vi "相机标定-汇川机械手.vi"() -> ()   [LabVIEW 2016]
uses:
  <vilib>/userdefined/High Color/IMAQdx.ctl
  CalibrateSteps.ctl
  <vilib>/vision/driver/IMAQdx.llb/IMAQdx Acquisition Mode.ctl
  <vilib>/vision/driver/IMAQdx.llb/IMAQdx Buffer Number Mode.ctl
  <vilib>/Utility/config.llb/Write Key (Boolean).vi
  <vilib>/vision/driver/NI_Vision_Acquisition_Software.lvlib
  <vilib>/Utility/config.llb/NI_LVConfig.lvlib
panel:
  in  "记录抓取位置":bool
  out "机械手抓取Y":dbl
  out "机械手抓取X":dbl
  out "连接成功":bool
  in  "重新连接":bool
  in  "X轴偏移量":dbl=10000.0
  in  "Y轴偏移量":dbl=10000.0
  in  "确定按钮":bool
  out "机械手坐标X":dbl
  out "机械手坐标Y":dbl
  out "像素坐标X":dbl
  out "像素坐标Y":dbl
  in  "强制退出":bool
  out "Image":T1(plugin-control)
  in  "CalibrationPath":path
  in  "SessionSelect":T2
  out "停止标志":bool
  # "影像显示"
  # "参数设置"
  # "结果显示"
  # "记录Mark位置"
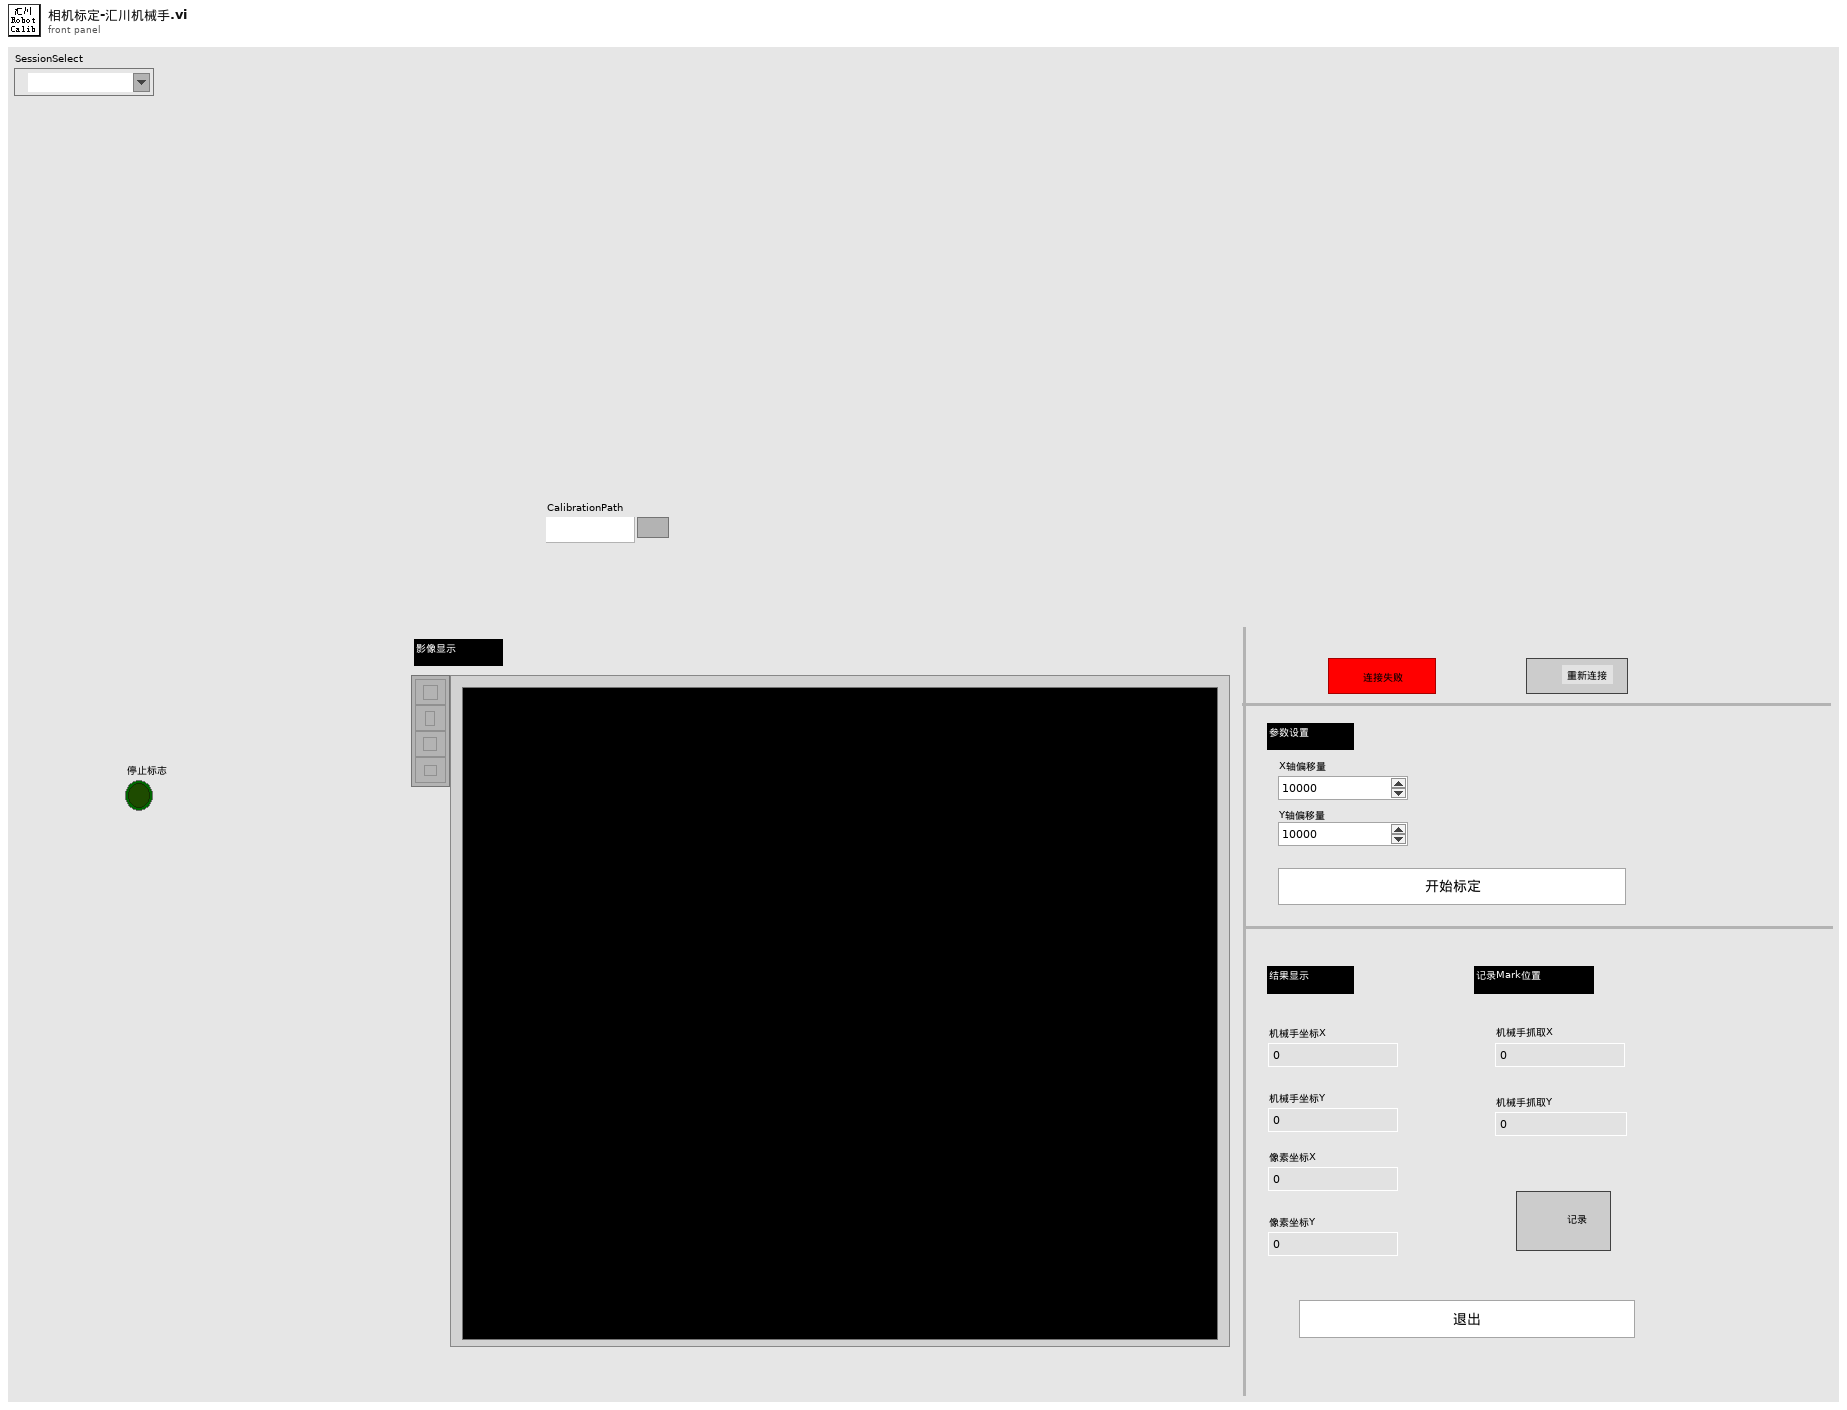
[diagram p1: front panel]
types:
  T1 = typedef "IMAQ Image.ctl" = refnum<image>
  T2 = typedef "IMAQdx.ctl" = refnum<k21>
  T3 = typedef "CalibrateSteps.ctl" = enum16{"初始化参数", "连接机械手", "连接相机", "机械手移动原位", "相机一次采集", "Y轴移动负偏移", "Y轴移动正偏移", "X轴移动正偏移", "X轴移动负偏移", "数据保存", "退出"}
  T4 = typedef "NI_LVConfig.lvlib/Config Data RefNum.ctl" = refnum<k1>
  T5 = enum16{"open", "replace", "create", "open or create", "replace or create", "replace or create with confirmation"}
  T6 = typedef "NI_Vision_Acquisition_Software.lvlib/IMAQdx Acquisition Mode.ctl" = enum32{"One Shot", "Continuous"}
  T7 = typedef "NI_Vision_Acquisition_Software.lvlib/IMAQdx Buffer Number Mode.ctl" = enum32{"Next", "Last", "Buffer Number", "Every", "Last New"}
  T8 = enum32{"Invalid", "Standard", "Closed", "Hidden", "Minimized", "Maximized"}
  T9 = cluster{"Center (Pixels)":cluster{"X":sgl, "Y":sgl}, "Radius (Pixels)":dbl, "Center (Real-World)":cluster{"X":sgl, "Y":sgl}, "Radius (Real-World)":dbl, "Roundness (Real-World)":dbl, "Average Strength":dbl, "Average SNR (dB)":dbl}
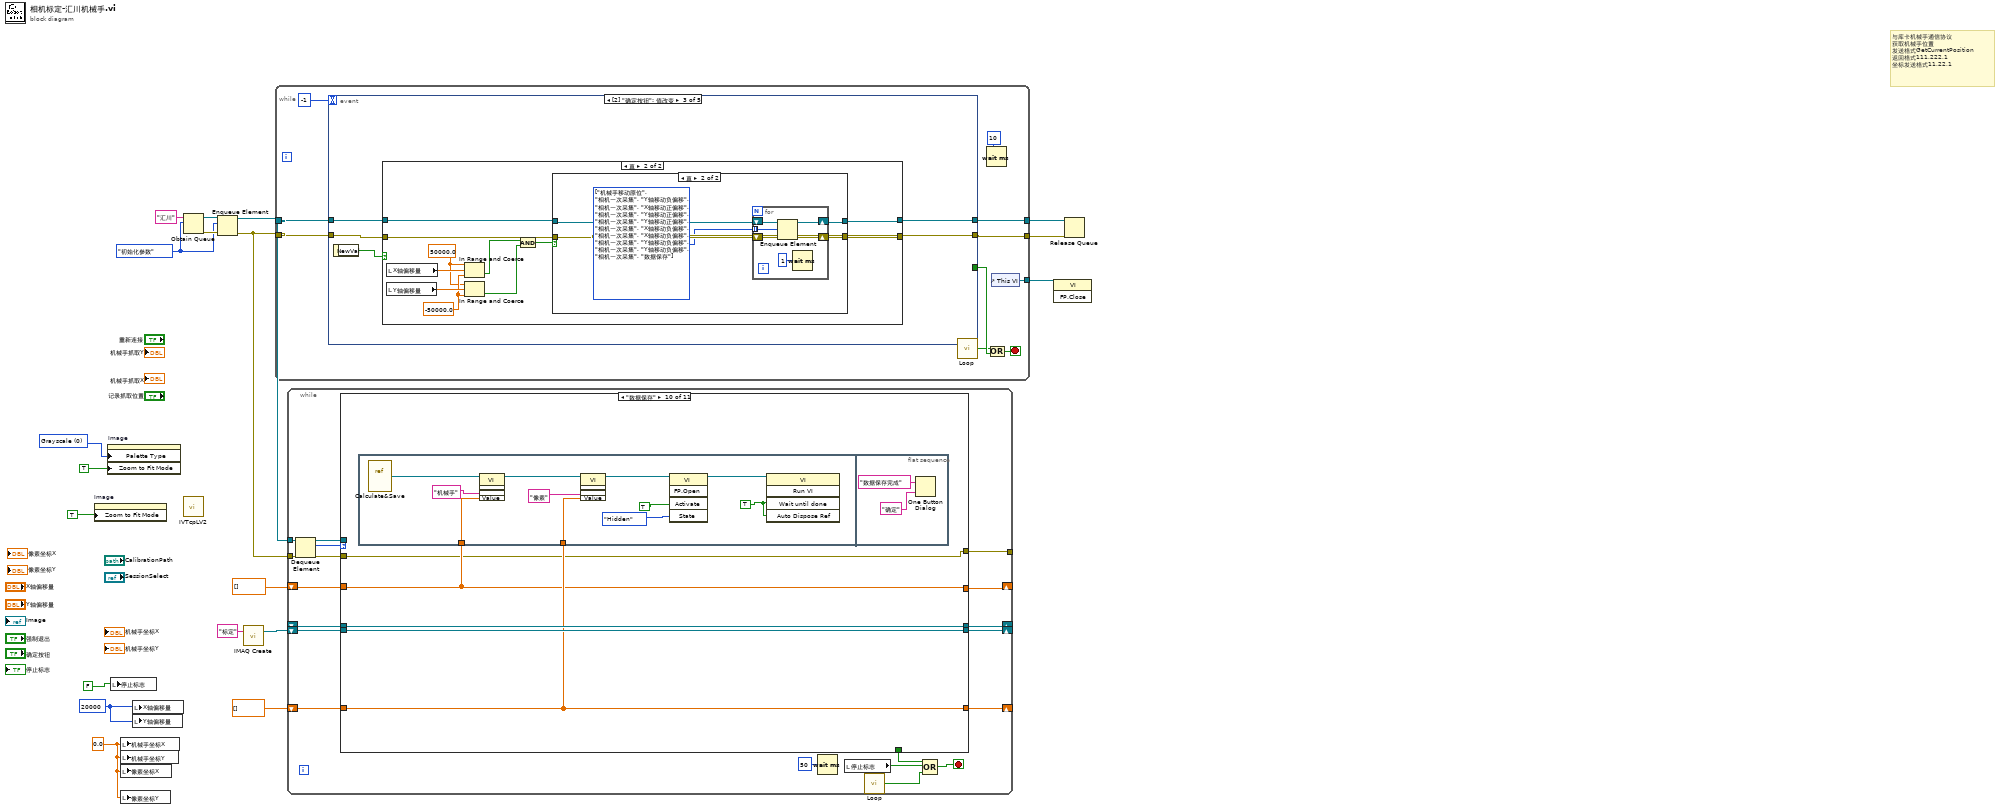
[diagram p0: block diagram]
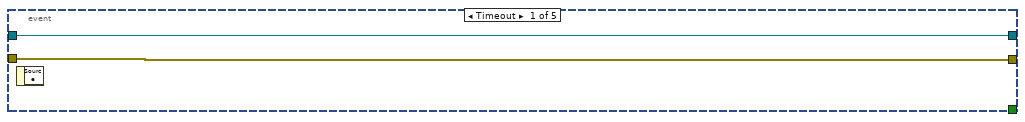
[diagram p2: hidden frame]
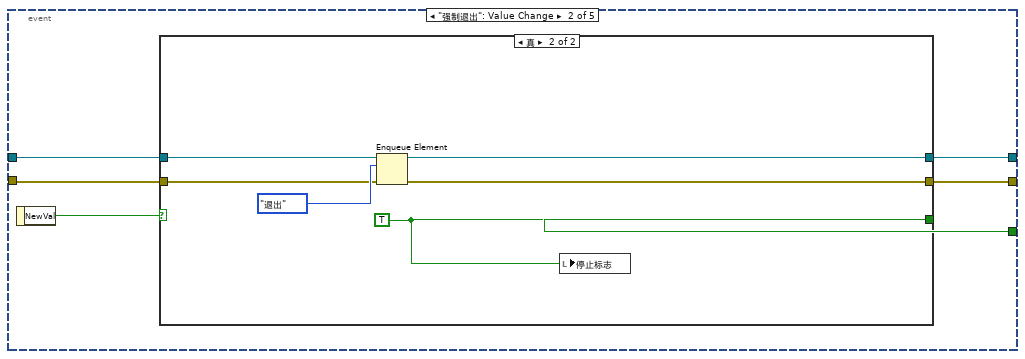
[diagram p3: hidden frame]
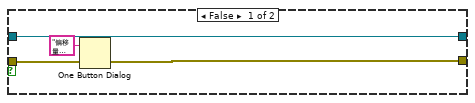
[diagram p6: hidden frame]
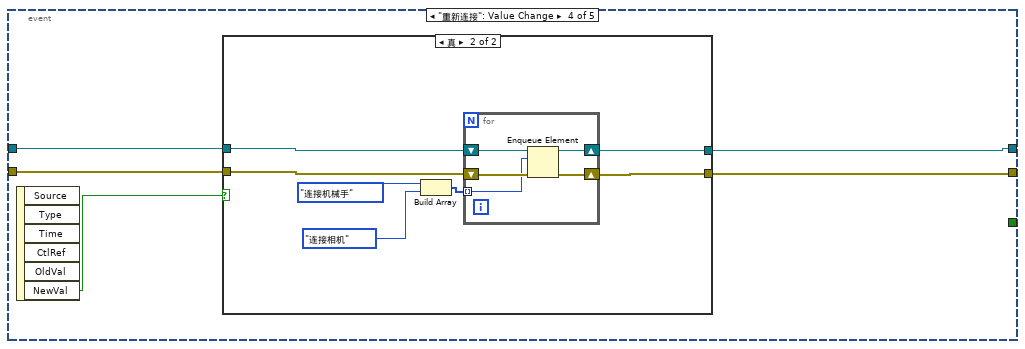
[diagram p7: hidden frame]
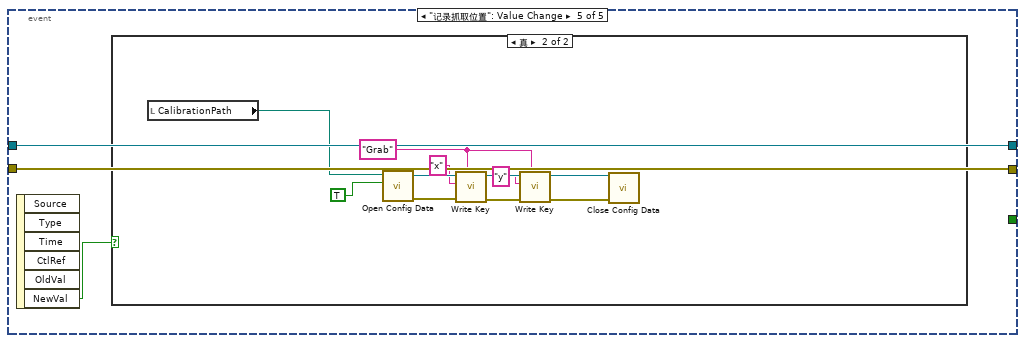
[diagram p9: hidden frame]
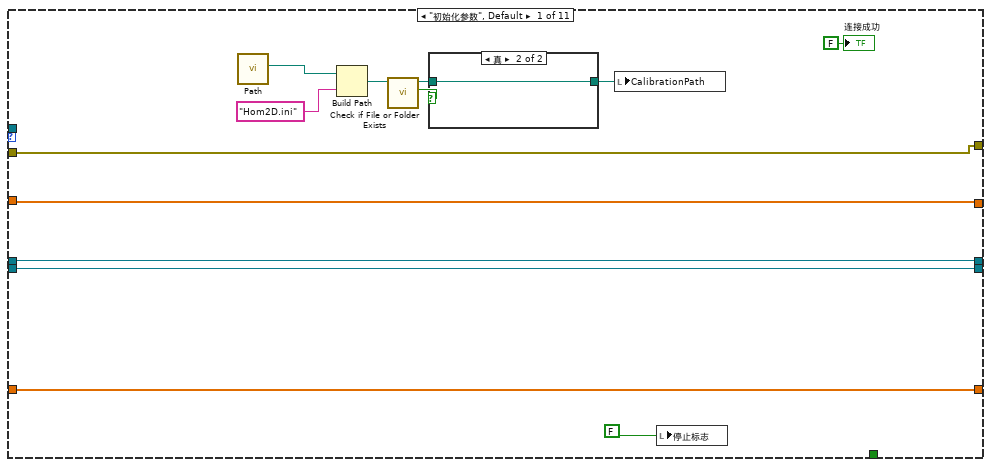
[diagram p11: hidden frame]
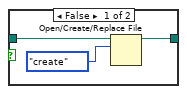
[diagram p12: hidden frame]
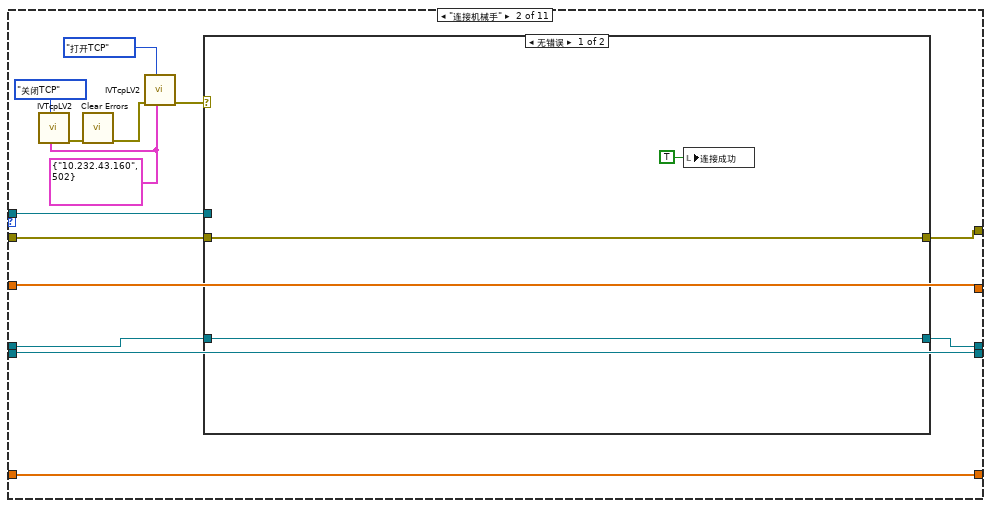
[diagram p13: hidden frame]
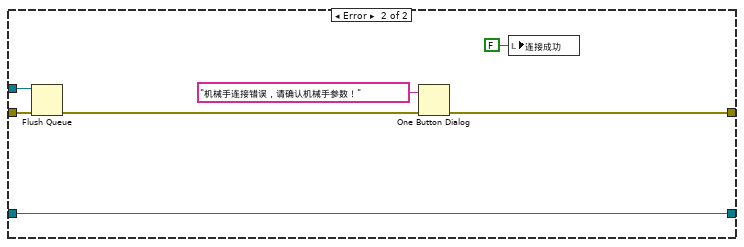
[diagram p14: hidden frame]
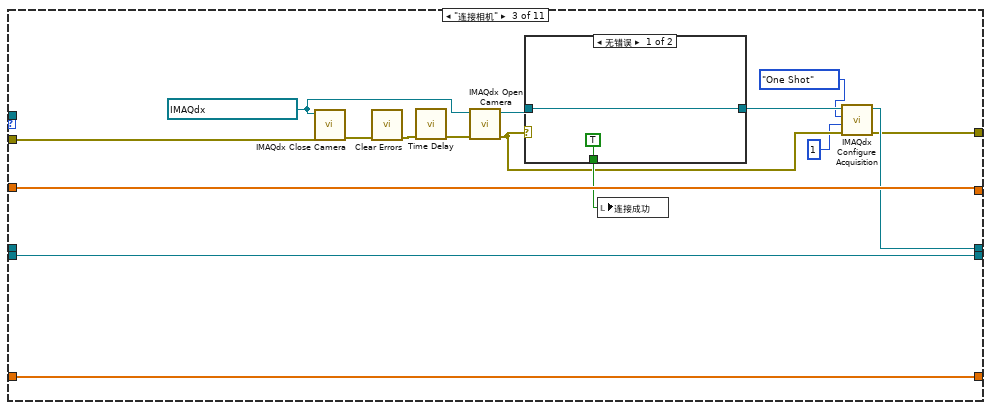
[diagram p15: hidden frame]
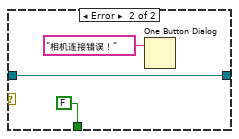
[diagram p16: hidden frame]
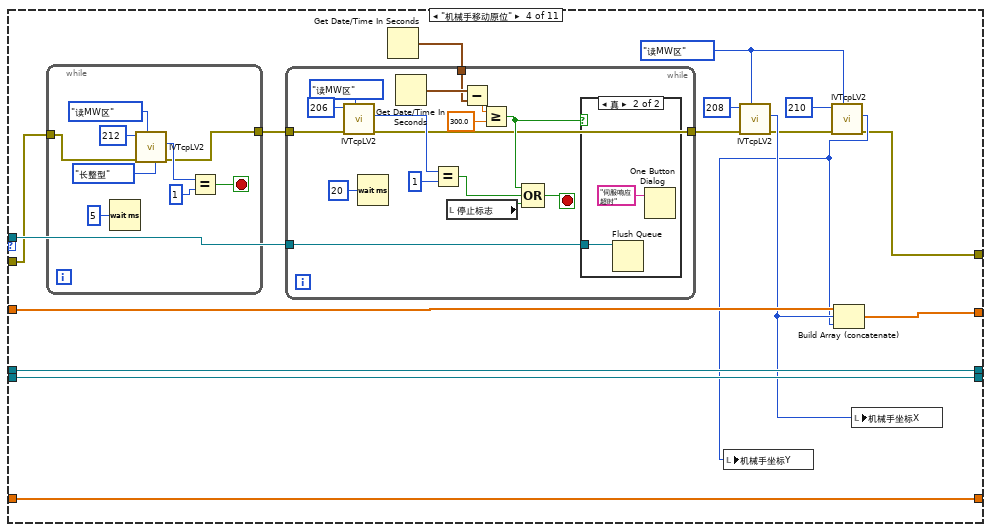
[diagram p17: hidden frame]
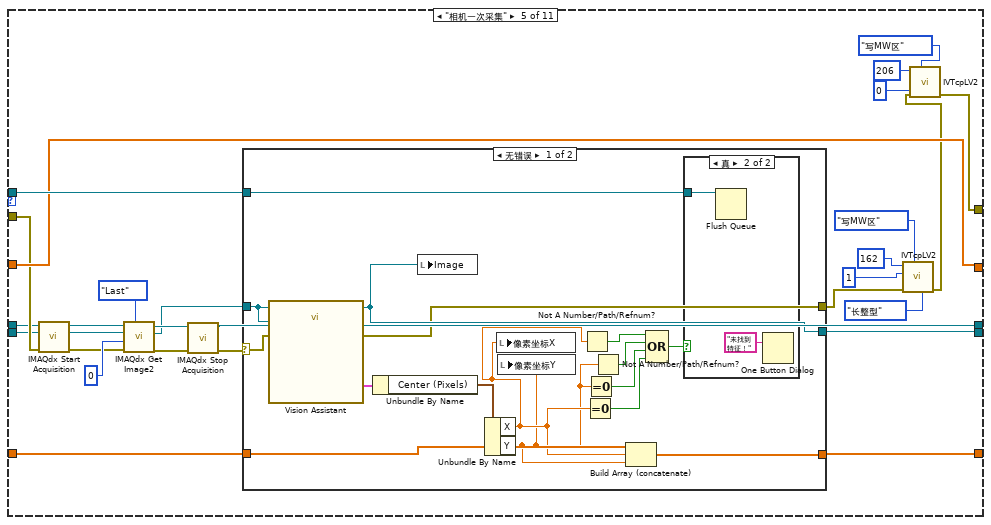
[diagram p19: hidden frame]
diagram:
  w3 = CalibrateSteps."初始化参数"
  w19 = 0.0 ("机械手当前X坐标")
  w16 = 20000
  w14 = u32 0 items=["Grayscale", "Binary", "Gradient", "Rainbow", "Temperature", "User Defined", "Binary 16 Bit", "Gradient 16 Bit", "Rainbow 16 Bit", "Temperature 16 Bit", "User Defined 16 Bit"] ("Palette:Palette Type")
  # "与库卡机械手通信协议\n获取机械手位置\n发送格式GetCurrentPosition\n返回格式111,222,1\n坐标发送格式11,22,1"
  n1 = property on="Image" class="ImageControl"("Zoom to Fit Mode"=TRUE) -> ()  [unwired: 2 in, 2 out]
  n2 = property on="Image" class="ImageControl"("Palette Type"=w14, "Zoom to Fit Mode"=TRUE) -> ()  [unwired: 2 in, 2 out]
  n3 = local write "停止标志"(FALSE ("停止标志")) -> ()
  n4 = local write "机械手坐标X"(w19) -> ()
  n5 = local write "机械手坐标Y"(w19) -> ()
  n6 = local write "像素坐标X"(w19) -> ()
  n7 = local write "像素坐标Y"(w19) -> ()
  n8 = local write "X轴偏移量"(w16) -> ()
  n9 = local write "Y轴偏移量"(w16) -> ()
  n10 = Obtain Queue(name (unnamed)="汇川", element data type=w3) -> (queue out=w6:refnum<queue>, error out=w5:errorcluster)  [unwired: 3 in, 1 out]
  n11 = call "IVTcpLV2.vi"() -> ()  [unwired: 8 in, 4 out]
  n12 = Enqueue Element(queue=w6, element=w3, error in (no error)=w5) -> (queue out=w4:refnum<queue>, error out=w2:errorcluster)  [unwired: 1 in, 1 out]
  n13 = call "IMAQ Create"("Image Name"="标定") -> ("New Image"=w8:T1)  [unwired: 4 in, 1 out]
  n14 = while {
    tunnel: w4 -> [w29]
    tunnel: w2 -> [w28]
    tunnel: [w27] -> w11
    tunnel: [w26] -> w12
    tunnel: [w24] -> w13
    stop <- w23 stop-if-true
    n15 = event shown="[2] \"确定按钮\": 值改变" {
      selector: _ -> [_ _ _ _ _]
      dyn-events: _ -> [_ _ _ _ _]
      timeout: -1 -> [_ _ _ _ _]
      tunnel: w29 -> [w31 w36 w49 w79 w98]
      tunnel: w28 -> [w30 w33 w48 w78 w97]
      tunnel: [w31 w35 w47 w81 w98] -> w27
      tunnel: [w30 w32 w46 w80 w97] -> w26
      tunnel: [_ w34 _ _ _] -> w22
      event Timeout {
        n16 = event-data() -> ()  [unwired: 1 in, 1 out]
      }
      event "强制退出": Value Change {
        n17 = event-data() -> ("NewVal"=w37:bool)  [unwired: 1 in]
        n18 = case shown="真" w37 {
          tunnel: [_ w43] -> w34
          tunnel: w36 -> [w39 w45]
          tunnel: [w39 w44] -> w35
          tunnel: w33 -> [w38 w41]
          tunnel: [w38 w40] -> w32
          frame False {
          }
          frame True {
            w43 = TRUE
            n19 = Enqueue Element(queue=w45, element=CalibrateSteps."退出", error in (no error)=w41) -> (queue out=w44:refnum<queue>, error out=w40:errorcluster)  [unwired: 1 in, 1 out]
            n20 = local write "停止标志"(w43) -> ()
          }
        }
      }
      event "确定按钮": Value Change {
        n21 = event-data() -> ("NewVal"=w50:bool)  [unwired: 1 in]
        n22 = case shown="真" w50 {
          tunnel: w49 -> [w52 w54]
          tunnel: w48 -> [w51 w53]
          tunnel: [w52 w56] -> w47
          tunnel: [w51 w55] -> w46
          frame False {
          }
          frame True {
            w58 = -50000.0 ("下限")
            w57 = 50000.0 ("上限")
            n23 = local read "Y轴偏移量"() -> (w60:dbl)
            n24 = local read "X轴偏移量"() -> (w59:dbl)
            n25 = In Range and Coerce(upper limit=w57, x=w60, lower limit=w58) -> (In Range?=w62:bool)  [unwired: 1 out]
            n26 = In Range and Coerce(upper limit=w57, x=w59, lower limit=w58) -> (In Range?=w61:bool)  [unwired: 1 out]
            n27 = And(x=w61, y=w62) -> (x .and. y?=w63:bool)
            n28 = case shown="真" w63 {
              tunnel: [w65 w71] -> w56
              tunnel: [w64 w70] -> w55
              tunnel: w54 -> [w65 w69]
              tunnel: w53 -> [w64 w68]
              frame False {
                n29 = One Button Dialog(message="偏移量设置太大请重新设置！" ("消息")) -> ()  [unwired: 1 in, 1 out]
              }
              frame True {
                w67 = T3[] [enum."机械手移动原位", enum."相机一次采集", enum."Y轴移动负偏移", enum."相机一次采集", enum."X轴移动正偏移", enum."相机一次采集", enum."Y轴移动正偏移", enum."相机一次采集", enum."Y轴移动正偏移", enum."相机一次采集", enum."X轴移动负偏移", enum."相机一次采集", enum."X轴移动负偏移", enum."相机一次采集", enum."Y轴移动负偏移", enum."相机一次采集", enum."Y轴移动负偏移", enum."相机一次采集", enum."数据保存"] items=["初始化参数", "连接机械手", "连接相机", "机械手移动原位", "相机一次采集", "Y轴移动负偏移", "Y轴移动正偏移", "X轴移动正偏移", "X轴移动负偏移", "数据保存", "退出"] ("Array")
                n30 = for {
                  shift-right: [w75] -> w71
                  shift-left: w69 -> [w77]
                  shift-right: [w74] -> w70
                  shift-left: w68 -> [w76]
                  tunnel: w67 -> [w73] mode=indexing
                  n31 = Enqueue Element(queue=w77, element=w73, error in (no error)=w76) -> (queue out=w75:refnum<queue>, error out=w74:errorcluster)  [unwired: 1 in, 1 out]
                  n32 = Wait (ms)(milliseconds to wait=u32 1 ("等待时间（毫秒）")) -> ()  [unwired: 1 out]
                }
              }
            }
          }
        }
      }
      event "重新连接": Value Change {
        n33 = event-data() -> ("NewVal"=w82:bool)  [unwired: 1 in, 5 out]
        n34 = case shown="真" w82 {
          tunnel: [w84 w91] -> w81
          tunnel: [w83 w90] -> w80
          tunnel: w79 -> [w84 w89]
          tunnel: w78 -> [w83 w88]
          frame False {
          }
          frame True {
            n35 = Build Array(CalibrateSteps."连接机械手", CalibrateSteps."连接相机") -> (w87:T3[])
            n36 = for {
              shift-right: [w94] -> w91
              shift-left: w89 -> [w96]
              shift-right: [w93] -> w90
              shift-left: w88 -> [w95]
              tunnel: w87 -> [w92] mode=indexing
              n37 = Enqueue Element(queue=w96, element=w92, error in (no error)=w95) -> (queue out=w94:refnum<queue>, error out=w93:errorcluster)  [unwired: 1 in, 1 out]
            }
          }
        }
      }
      event "记录抓取位置": Value Change {
        n38 = event-data() -> ("NewVal"=w99:bool)  [unwired: 1 in, 5 out]
        n39 = case shown="真" w99 {
          frame False {
          }
          frame True {
            w105 = "Grab" ("key")
            n40 = local read "CalibrationPath"() -> (w102:path)
            n41 = call <vilib>:"Open Config Data.vi"("create file if necessary (T)"=TRUE, "configuration file path"=w102) -> ("error out"=w108:errorcluster, "refnum"=w110:T4)  [unwired: 7 in, 1 out]
            n42 = call-poly <vilib>:"Write Key.vi"("section"=w105, "error in (no error)"=w108, "key"="x", "refnum"=w110) -> ("error out"=w107:errorcluster, "refnum out"=w106:T4)  [unwired: 5 in, 1 out]
            n43 = call-poly <vilib>:"Write Key.vi"("section"=w105, "error in (no error)"=w107, "key"="y", "refnum"=w106) -> ("error out"=w100:errorcluster, "refnum out"=w101:T4)  [unwired: 5 in, 1 out]
            n44 = call <vilib>:"Close Config Data.vi"("error in (no error)"=w100, "refnum"=w101) -> ()  [unwired: 8 in, 2 out]
          }
        }
      }
    }
    n45 = call "Loop.vi"() -> ("Loop Out"=w21:bool)  [unwired: 5 in]
    n46 = Wait (ms)(milliseconds to wait=u32 10 ("等待时间（毫秒）")) -> ()  [unwired: 1 out]
    n47 = Compound Arithmetic op=OR ("复合运算")(w21, w22) -> (w23:bool)
    n48 = control-ref of="This VI"() -> (w24:refnum<vi>)
  }
  n49 = while {
    shift-right: [w126] -> _
    shift-left: dbl[] [] -> [w125]
    shift-right: [w116] -> _
    shift-left: dbl[] [] -> [w112]
    shift-right: [w123] -> _
    shift-left: _ -> [w122]
    shift-right: [w120] -> _
    shift-left: w8 -> [w121]
    tunnel: w4 -> [w119]
    tunnel: w2 -> [w115]
    tunnel: [w113] -> _
    stop <- w127 stop-if-true
    n50 = Dequeue Element(queue=w119, error in (no error)=w115) -> (queue out=w117:refnum<queue>, element=w118:T3, error out=w114:errorcluster)  [unwired: 1 in, 1 out]
    n51 = case shown="\"数据保存\"" w118 {
      tunnel: w112 -> [w139 w155 w184 w206 w256 w309 w346 w390 w432 w455 w472]
      tunnel: [w139 w155 w184 w204 w256 w306 w345 w389 w431 w455 w472] -> w116
      tunnel: [w142 w159 w169 w205 w260 w310 w344 w385 w427 w456 w477] -> w126
      tunnel: w125 -> [w142 w159 w169 w205 w259 w310 w344 w385 w427 w456 w477]
      tunnel: [_ _ _ _ _ _ _ _ _ _ TRUE] -> w124
      tunnel: [w141 w158 w173 w203 w249 w308 w352 w394 w436 w458 w476] -> w123
      tunnel: w122 -> [w141 w157 _ w203 w246 w308 w352 w394 w436 w458 w476]
      tunnel: [w140 w156 w183 w202 w258 w307 w351 w393 w435 w457 w475] -> w120
      tunnel: w121 -> [w140 w156 w183 w202 w251 w307 w351 w393 w435 w457 w475]
      tunnel: w117 -> [_ w154 _ w200 w257 w303 w348 w388 w430 _ _]
      tunnel: w114 -> [w131 w153 w175 w199 w253 w295 w347 w378 w420 w454 w473]
      tunnel: [w131 w152 w172 w190 w235 w293 w347 w377 w420 w454 w473] -> w113
      frame "初始化参数", Default {
        n52 = call "Path.vi"() -> ("Total"=w130:path)  [unwired: 11 in]
        n53 = Build Path(base path=w130, name or relative path="Hom2D.ini") -> (appended path=w136:path)
        n54 = call <vilib>:"Check if File or Folder Exists.vi"("path"=w136) -> ("file or folder exists?"=w138:bool, "dup path"=w137:path)  [unwired: 8 in, 1 out]
        n55 = case shown="真" w138 {
          tunnel: w137 -> [w144 w145]
          tunnel: [w144 w145] -> w135
          frame False {
            n56 = Open/Create/Replace File(file path (use dialog)=w144, operation (0:open)=T5."create") -> ()  [unwired: 4 in, 3 out]
          }
          frame True {
          }
        }
        n57 = local write "CalibrationPath"(w135) -> ()
        n58 = local write "停止标志"(FALSE ("停止标志")) -> ()
        "连接成功" <- FALSE ("连接成功")
      }
      frame "连接机械手" {
        w146 = cluster{"IP地址":string, "端口":u16} {"IP地址"="10.232.43.160", "端口"=502} ("TCP连接参数")
        n59 = call "IVTcpLV2.vi"("TCP连接参数"=w146, "TCP操作模式"=enum16{"打开TCP", "读MW区", "写MW区", "关闭TCP"}."关闭TCP") -> ("错误输出"=w147:errorcluster)  [unwired: 6 in, 3 out]
        n60 = call <vilib>:"Clear Errors.vi"("error in (no error)"=w147) -> ("error out"=w151:errorcluster)  [unwired: 5 in, 1 out]
        n61 = call "IVTcpLV2.vi"("TCP连接参数"=w146, "TCP操作模式"=enum16{"打开TCP", "读MW区", "写MW区", "关闭TCP"}."打开TCP", "错误输入"=w151) -> ("错误输出"=w150:errorcluster)  [unwired: 5 in, 3 out]
        n62 = case shown="无错误" w150 {
          tunnel: [w162 w168] -> w158
          tunnel: w157 -> [w162 w168]
          tunnel: w154 -> [_ w166]
          tunnel: w153 -> [w160 w164]
          tunnel: [w160 w163] -> w152
          frame No Error {
            n63 = local write "连接成功"(TRUE ("连接成功")) -> ()
          }
          frame Error {
            n64 = Flush Queue(queue=w166, error in (no error)=w164) -> (error out=w163:errorcluster)  [unwired: 2 out]
            n65 = One Button Dialog(message="机械手连接错误，请确认机械手参数！") -> ()  [unwired: 1 in, 1 out]
            n66 = local write "连接成功"(FALSE ("连接成功")) -> ()
          }
        }
      }
      frame "连接相机" {
        w177 = T2 "MV-CA060-11GM" ("Session In")
        n67 = call <vilib>:"IMAQdx Close Camera.vi"("error in"=w175, "Session In"=w177) -> ("error out"=w182:errorcluster)  [unwired: 9 in]
        n68 = call <vilib>:"Clear Errors.vi"("error in (no error)"=w182) -> ("error out"=w181:errorcluster)  [unwired: 5 in, 1 out]
        n69 = call "Time Delay"("error in (no error)"=w181) -> ("error out"=w180:errorcluster)  [unwired: 10 in]
        n70 = call <vilib>:"IMAQdx Open Camera.vi"("error in"=w180, "Session In"=w177) -> ("error out"=w174:errorcluster, "Session Out"=w179:T2)  [unwired: 8 in]
        n71 = case shown="无错误" w174 {
          tunnel: w179 -> [w186 w189]
          tunnel: [w186 w189] -> w176
          tunnel: [TRUE ("连接成功") FALSE ("连接成功")] -> w178
          frame No Error {
          }
          frame Error {
            n72 = One Button Dialog(message="相机连接错误！") -> ()  [unwired: 1 in, 1 out]
          }
        }
        n73 = local write "连接成功"(w178) -> ()
        n74 = call <vilib>:"IMAQdx Configure Acquisition.vi"("error in"=w174, "Number of Buffers"=u32 1, "Continuous?"=IMAQdx_Acquisition_Mode."One Shot", "Session In"=w176) -> ("error out"=w172:errorcluster, "Session Out"=w173:T2)  [unwired: 6 in]
      }
      frame "机械手移动原位" {
        w193 = enum16{"打开TCP", "读MW区", "写MW区", "关闭TCP"}."读MW区" ("TCP操作模式")
        n75 = while {
          tunnel: w199 -> [w212]
          tunnel: [w207] -> w198
          stop <- w210 stop-if-true
          n76 = Wait (ms)(milliseconds to wait=u32 5 ("等待时间（毫秒）")) -> ()  [unwired: 1 out]
          n77 = call "IVTcpLV2.vi"("数值类型"=enum16{"长整型", "双精度"}."长整型", "TCP操作模式"=enum16{"打开TCP", "读MW区", "写MW区", "关闭TCP"}."读MW区", "错误输入"=w212, "寄存器MD地址"=212) -> ("错误输出"=w207:errorcluster, "数值"=w211:u32)  [unwired: 4 in, 2 out]
          n78 = Equal?(x=w211, y=1) -> (x = y?=w210:bool)
        }
        n79 = Get Date/Time In Seconds() -> (seconds since 1Jan1904=w201:timestamp)
        n80 = while {
          tunnel: w198 -> [w223]
          tunnel: w201 -> [w226]
          tunnel: w200 -> [w224]
          tunnel: [w216] -> w197
          stop <- w231 stop-if-true
          n81 = call "IVTcpLV2.vi"("TCP操作模式"=enum16{"打开TCP", "读MW区", "写MW区", "关闭TCP"}."读MW区", "错误输入"=w223, "寄存器MD地址"=206) -> ("错误输出"=w216:errorcluster, "数值"=w219:u32)  [unwired: 5 in, 2 out]
          n82 = Wait (ms)(milliseconds to wait=u32 20 ("等待时间（毫秒）")) -> ()  [unwired: 1 out]
          n83 = Get Date/Time In Seconds() -> (seconds since 1Jan1904=w228:timestamp)
          n84 = Equal?(x=w219, y=u32 1) -> (x = y?=w217:bool)
          n85 = local read "停止标志"() -> (w230:bool)
          n86 = Subtract(x=w228, y=w226) -> (x-y=w229:dbl)
          n87 = Greater Or Equal?(x=w229, y=300.0) -> (x >= y?=w225:bool)
          n88 = Compound Arithmetic op=OR(w225, w217, w230) -> (w231:bool)
          n89 = case shown="真" w225 {
            tunnel: w224 -> [_ w232]
            frame False {
            }
            frame True {
              n90 = Flush Queue(queue=w232) -> ()  [unwired: 1 in, 3 out]
              n91 = One Button Dialog(message="伺服响应超时") -> ()  [unwired: 1 in, 1 out]
            }
          }
        }
        n92 = call "IVTcpLV2.vi"("TCP操作模式"=w193, "错误输入"=w197, "寄存器MD地址"=208) -> ("错误输出"=w194:errorcluster, "数值"=w195:u32)  [unwired: 5 in, 2 out]
        n93 = call "IVTcpLV2.vi"("TCP操作模式"=w193, "错误输入"=w194, "寄存器MD地址"=210) -> ("错误输出"=w190:errorcluster, "数值"=w191:u32)  [unwired: 5 in, 2 out]
        n94 = local write "机械手坐标Y"(w191) -> ()
        n95 = Build Array (concatenate)(w206, w195, w191) -> (w204:dbl[])
        n96 = local write "机械手坐标X"(w195) -> ()
      }
      frame "相机一次采集" {
        n97 = call <vilib>:"IMAQdx Start Acquisition.vi"("error in"=w253, "Session In"=w246) -> ("error out"=w247:errorcluster, "Session Out"=w252:T2)  [unwired: 8 in]
        n98 = call <vilib>:"IMAQdx Get Image2.vi"("Buffer Number Mode (Next)"=IMAQdx_Buffer_Number_Mode."Last", "error in"=w247, "Buffer Number In"=u32 0, "Image In"=w251, "Session In"=w252) -> ("error out"=w248:errorcluster, "Image Out"=w244:T1, "Session Out"=w250:T2)  [unwired: 3 in, 1 out]
        n99 = call <vilib>:"IMAQdx Stop Acquisition.vi"("error in"=w248, "Session In"=w250) -> ("error out"=w245:errorcluster, "Session Out"=w249:T2)  [unwired: 8 in]
        n100 = case shown="无错误" w245 {
          selector: w245 -> [w262 w279]
          tunnel: [w276 w285] -> w260
          tunnel: w259 -> [w275 w285]
          tunnel: [w263 w281] -> w258
          tunnel: w257 -> [w271 w282]
          tunnel: w244 -> [w268 w281]
          tunnel: [w261 w280] -> w243
          frame No Error {
            n101 = call "Vision Assistant"("Image In"=w268, "Image Dst"=w268, "error in"=w262) -> ("Image Out"=w263:T1, "Fitted Circle (Find Circular Edge 1)"=w267:T9, "error out"=w261:errorcluster)  [unwired: 22 in]
            n102 = Unbundle By Name(w267) -> ("Center (Pixels)"=w266:cluster{"X":sgl, "Y":sgl})
            n103 = local write "Image"(w263) -> ()
            n104 = Unbundle By Name(w266) -> ("X"=w265:sgl, "Y"=w264:sgl)
            n105 = local write "像素坐标X"(w265) -> ()
            n106 = local write "像素坐标Y"(w264) -> ()
            n107 = Not A Number/Path/Refnum?(number/path/refnum=w265) -> (NaN/Path/Refnum?=w273:bool)
            n108 = Equal To 0?(x=w265) -> (x = 0?=w269:bool)
            n109 = Equal To 0?(x=w264) -> (x = 0?=w270:bool)
            n110 = Not A Number/Path/Refnum?(number/path/refnum=w264) -> (NaN/Path/Refnum?=w272:bool)
            n111 = Build Array (concatenate)(w275, w265, w264) -> (w276:dbl[])
            n112 = Compound Arithmetic op=OR(w273, w272, w270, w269) -> (w274:bool)
            n113 = case shown="真" w274 {
              tunnel: w271 -> [_ w277]
              frame False {
              }
              frame True {
                n114 = Flush Queue(queue=w277) -> ()  [unwired: 1 in, 3 out]
                n115 = One Button Dialog(message="未找到特征！") -> ()  [unwired: 1 in, 1 out]
              }
            }
          }
          frame Error {
            n116 = Flush Queue(queue=w282) -> ()  [unwired: 1 in, 3 out]
            n117 = One Button Dialog(message="相机出错，检查相机连接！" ("消息"), button name ("OK")="确定" ("按钮名称（“确定”）")) -> ()  [unwired: 1 out]
            n118 = call <vilib>:"Clear Errors.vi"("error in (no error)"=w279) -> ("error out"=w280:errorcluster)  [unwired: 5 in, 1 out]
          }
        }
        n119 = call "IVTcpLV2.vi"("数值类型"=enum16{"长整型", "双精度"}."长整型", "TCP操作模式"=enum16{"打开TCP", "读MW区", "写MW区", "关闭TCP"}."写MW区", "错误输入"=w243, "值"=1, "寄存器MD地址"=162) -> ("错误输出"=w236:errorcluster)  [unwired: 3 in, 3 out]
        n120 = call "IVTcpLV2.vi"("TCP操作模式"=enum16{"打开TCP", "读MW区", "写MW区", "关闭TCP"}."写MW区", "错误输入"=w236, "值"=0, "寄存器MD地址"=206) -> ("错误输出"=w235:errorcluster)  [unwired: 4 in, 3 out]
      }
      frame "Y轴移动负偏移" {
        w291 = enum16{"打开TCP", "读MW区", "写MW区", "关闭TCP"}."写MW区" ("TCP操作模式")
        n121 = local read "机械手坐标X"() -> (w300:dbl)
        n122 = local read "机械手坐标Y"() -> (w302:dbl)
        n123 = local read "Y轴偏移量"() -> (w301:dbl)
        n124 = Subtract(x=w302, y=w301) -> (x-y=w299:dbl)
        n125 = Multiply(x=w301, y=-1.0) -> (x*y=w297:dbl)
        n126 = call "IVTcpLV2.vi"("TCP操作模式"=w291, "错误输入"=w295, "值"=w297, "寄存器MD地址"=138) -> ("错误输出"=w292:errorcluster)  [unwired: 4 in, 3 out]
        n127 = call "IVTcpLV2.vi"("TCP操作模式"=w291, "错误输入"=w292, "值"=0, "寄存器MD地址"=136) -> ("错误输出"=w288:errorcluster)  [unwired: 4 in, 3 out]
        n128 = local write "机械手坐标X"(w300) -> ()
        n129 = local write "机械手坐标Y"(w299) -> ()
        n130 = call "Time Delay3"("error in (no error)"=w288) -> ("error out"=w286:errorcluster)  [unwired: 10 in]
        n131 = call "IVTcpLV2.vi"("TCP操作模式"=w291, "错误输入"=w286, "值"=1, "寄存器MD地址"=160) -> ("错误输出"=w287:errorcluster)  [unwired: 4 in, 3 out]
        n132 = Get Date/Time In Seconds() -> (seconds since 1Jan1904=w304:timestamp)
        n133 = while {
          tunnel: w287 -> [w317]
          tunnel: w304 -> [w320]
          tunnel: w303 -> [w318]
          tunnel: [w311] -> w293
          stop <- w326 stop-if-true
          n134 = call "IVTcpLV2.vi"("TCP操作模式"=enum16{"打开TCP", "读MW区", "写MW区", "关闭TCP"}."读MW区", "错误输入"=w317, "寄存器MD地址"=206) -> ("错误输出"=w311:errorcluster, "数值"=w314:u32)  [unwired: 5 in, 2 out]
          n135 = Equal?(x=w314, y=u32 1) -> (x = y?=w312:bool)
          n136 = local read "停止标志"() -> (w324:bool)
          n137 = Wait (ms)(milliseconds to wait=u32 20 ("等待时间（毫秒）")) -> ()  [unwired: 1 out]
          n138 = Get Date/Time In Seconds() -> (seconds since 1Jan1904=w322:timestamp)
          n139 = Subtract(x=w322, y=w320) -> (x-y=w323:dbl)
          n140 = Greater Or Equal?(x=w323, y=300.0) -> (x >= y?=w319:bool)
          n141 = Compound Arithmetic op=OR(w319, w312, w324) -> (w326:bool)
          n142 = case shown="假" w319 {
            tunnel: w318 -> [_ w327]
            frame False {
            }
            frame True {
              n143 = Flush Queue(queue=w327) -> ()  [unwired: 1 in, 3 out]
              n144 = One Button Dialog(message="机械手响应超时") -> ()  [unwired: 1 in, 1 out]
            }
          }
        }
        n145 = Build Array (concatenate)(w309, w300, w299) -> (w306:dbl[])
      }
      frame "Y轴移动正偏移" {
        w334 = enum16{"打开TCP", "读MW区", "写MW区", "关闭TCP"}."写MW区" ("TCP操作模式")
        n146 = local read "机械手坐标Y"() -> (w343:dbl)
        n147 = local read "机械手坐标X"() -> (w341:dbl)
        n148 = local read "Y轴偏移量"() -> (w342:dbl)
        n149 = Add(x=w343, y=w342) -> (x+y=w340:dbl)
        n150 = Multiply(x=w342, y=1.0) -> (x*y=w336:dbl)
        n151 = call "IVTcpLV2.vi"("TCP操作模式"=w334, "值"=w336, "寄存器MD地址"=138) -> ("错误输出"=w335:errorcluster)  [unwired: 5 in, 3 out]
        n152 = local write "机械手坐标X"(w341) -> ()
        n153 = local write "机械手坐标Y"(w340) -> ()
        n154 = call "IVTcpLV2.vi"("TCP操作模式"=w334, "错误输入"=w335, "值"=0, "寄存器MD地址"=136) -> ("错误输出"=w330:errorcluster)  [unwired: 4 in, 3 out]
        n155 = call "Time Delay4"("error in (no error)"=w330) -> ("error out"=w329:errorcluster)  [unwired: 10 in]
        n156 = call "IVTcpLV2.vi"("TCP操作模式"=w334, "错误输入"=w329, "值"=1, "寄存器MD地址"=160) -> ("错误输出"=w331:errorcluster)  [unwired: 4 in, 3 out]
        n157 = Get Date/Time In Seconds() -> (seconds since 1Jan1904=w349:timestamp)
        n158 = while {
          tunnel: w331 -> [w356]
          tunnel: w349 -> [w361]
          tunnel: w348 -> [w359]
          stop <- w367 stop-if-true
          n159 = call "IVTcpLV2.vi"("TCP操作模式"=enum16{"打开TCP", "读MW区", "写MW区", "关闭TCP"}."读MW区", "错误输入"=w356, "寄存器MD地址"=206) -> ("数值"=w355:u32)  [unwired: 5 in, 3 out]
          n160 = Wait (ms)(milliseconds to wait=u32 20 ("等待时间（毫秒）")) -> ()  [unwired: 1 out]
          n161 = Equal?(x=w355, y=u32 1) -> (x = y?=w354:bool)
          n162 = local read "停止标志"() -> (w365:bool)
          n163 = Get Date/Time In Seconds() -> (seconds since 1Jan1904=w363:timestamp)
          n164 = Subtract(x=w363, y=w361) -> (x-y=w364:dbl)
          n165 = Greater Or Equal?(x=w364, y=300.0) -> (x >= y?=w360:bool)
          n166 = Compound Arithmetic op=OR(w360, w354, w365) -> (w367:bool)
          n167 = case shown="真" w360 {
            tunnel: w359 -> [_ w368]
            frame False {
            }
            frame True {
              n168 = Flush Queue(queue=w368) -> ()  [unwired: 1 in, 3 out]
              n169 = One Button Dialog(message="机械手响应超时") -> ()  [unwired: 1 in, 1 out]
            }
          }
        }
        n170 = Build Array (concatenate)(w346, w341, w340) -> (w345:dbl[])
      }
      frame "X轴移动正偏移" {
        w375 = enum16{"打开TCP", "读MW区", "写MW区", "关闭TCP"}."写MW区" ("TCP操作模式")
        n171 = local read "机械手坐标Y"() -> (w383:dbl)
        n172 = local read "机械手坐标X"() -> (w387:dbl)
        n173 = local read "X轴偏移量"() -> (w386:dbl)
        n174 = Add(x=w386, y=w387) -> (x+y=w384:dbl)
        n175 = Multiply(x=w386, y=1.0) -> (x*y=w379:dbl)
        n176 = call "IVTcpLV2.vi"("TCP操作模式"=w375, "错误输入"=w378, "值"=w379, "寄存器MD地址"=136) -> ("错误输出"=w376:errorcluster)  [unwired: 4 in, 3 out]
        n177 = call "IVTcpLV2.vi"("TCP操作模式"=w375, "错误输入"=w376, "值"=0, "寄存器MD地址"=138) -> ("错误输出"=w371:errorcluster)  [unwired: 4 in, 3 out]
        n178 = call "Time Delay6"("error in (no error)"=w371) -> ("error out"=w370:errorcluster)  [unwired: 10 in]
        n179 = local write "机械手坐标X"(w384) -> ()
        n180 = local write "机械手坐标Y"(w383) -> ()
        n181 = call "IVTcpLV2.vi"("TCP操作模式"=w375, "错误输入"=w370, "值"=1, "寄存器MD地址"=160) -> ("错误输出"=w372:errorcluster)  [unwired: 4 in, 3 out]
        n182 = Get Date/Time In Seconds() -> (seconds since 1Jan1904=w391:timestamp)
        n183 = while {
          tunnel: w372 -> [w399]
          tunnel: w391 -> [w404]
          tunnel: w388 -> [w402]
          tunnel: [w395] -> w377
          stop <- w410 stop-if-true
          n184 = call "IVTcpLV2.vi"("TCP操作模式"=enum16{"打开TCP", "读MW区", "写MW区", "关闭TCP"}."读MW区", "错误输入"=w399, "寄存器MD地址"=206) -> ("错误输出"=w395:errorcluster, "数值"=w398:u32)  [unwired: 5 in, 2 out]
          n185 = Wait (ms)(milliseconds to wait=u32 20 ("等待时间（毫秒）")) -> ()  [unwired: 1 out]
          n186 = Equal?(x=w398, y=u32 1) -> (x = y?=w397:bool)
          n187 = local read "停止标志"() -> (w408:bool)
          n188 = Get Date/Time In Seconds() -> (seconds since 1Jan1904=w406:timestamp)
          n189 = Subtract(x=w406, y=w404) -> (x-y=w407:dbl)
          n190 = Greater Or Equal?(x=w407, y=300.0) -> (x >= y?=w403:bool)
          n191 = Compound Arithmetic op=OR(w403, w397, w408) -> (w410:bool)
          n192 = case shown="真" w403 {
            tunnel: w402 -> [_ w411]
            frame False {
            }
            frame True {
              n193 = Flush Queue(queue=w411) -> ()  [unwired: 1 in, 3 out]
              n194 = One Button Dialog(message="机械手响应超时") -> ()  [unwired: 1 in, 1 out]
            }
          }
        }
        n195 = Build Array (concatenate)(w390, w384, w383) -> (w389:dbl[])
      }
      frame "X轴移动负偏移" {
        w418 = enum16{"打开TCP", "读MW区", "写MW区", "关闭TCP"}."写MW区" ("TCP操作模式")
        n196 = local read "机械手坐标Y"() -> (w425:dbl)
        n197 = local read "机械手坐标X"() -> (w428:dbl)
        n198 = local read "X轴偏移量"() -> (w429:dbl)
        n199 = Subtract(x=w428, y=w429) -> (x-y=w426:dbl)
        n200 = Multiply(x=w429, y=-1.0) -> (x*y=w421:dbl)
        n201 = call "IVTcpLV2.vi"("TCP操作模式"=w418, "错误输入"=w420, "值"=w421, "寄存器MD地址"=136) -> ("错误输出"=w419:errorcluster)  [unwired: 4 in, 3 out]
        n202 = local write "机械手坐标X"(w426) -> ()
        n203 = local write "机械手坐标Y"(w425) -> ()
        n204 = call "IVTcpLV2.vi"("TCP操作模式"=w418, "错误输入"=w419, "值"=0, "寄存器MD地址"=138) -> ("错误输出"=w415:errorcluster)  [unwired: 4 in, 3 out]
        n205 = call "Time Delay7"("error in (no error)"=w415) -> ("error out"=w414:errorcluster)  [unwired: 10 in]
        n206 = call "IVTcpLV2.vi"("TCP操作模式"=w418, "错误输入"=w414, "值"=1, "寄存器MD地址"=160) -> ("错误输出"=w413:errorcluster)  [unwired: 4 in, 3 out]
        n207 = Get Date/Time In Seconds() -> (seconds since 1Jan1904=w433:timestamp)
        n208 = while {
          tunnel: w413 -> [w440]
          tunnel: w433 -> [w445]
          tunnel: w430 -> [w443]
          stop <- w451 stop-if-true
          n209 = call "IVTcpLV2.vi"("TCP操作模式"=enum16{"打开TCP", "读MW区", "写MW区", "关闭TCP"}."读MW区", "错误输入"=w440, "寄存器MD地址"=206) -> ("数值"=w439:u32)  [unwired: 5 in, 3 out]
          n210 = Wait (ms)(milliseconds to wait=u32 20 ("等待时间（毫秒）")) -> ()  [unwired: 1 out]
          n211 = local read "停止标志"() -> (w449:bool)
          n212 = Equal?(x=w439, y=u32 1) -> (x = y?=w437:bool)
          n213 = Get Date/Time In Seconds() -> (seconds since 1Jan1904=w447:timestamp)
          n214 = Subtract(x=w447, y=w445) -> (x-y=w448:dbl)
          n215 = Greater Or Equal?(x=w448, y=300.0) -> (x >= y?=w444:bool)
          n216 = Compound Arithmetic op=OR(w444, w437, w449) -> (w451:bool)
          n217 = case shown="真" w444 {
            tunnel: w443 -> [_ w452]
            frame False {
            }
            frame True {
              n218 = Flush Queue(queue=w452) -> ()  [unwired: 1 in, 3 out]
              n219 = One Button Dialog(message="机械手响应超时") -> ()  [unwired: 1 in, 1 out]
            }
          }
        }
        n220 = Build Array (concatenate)(w432, w426, w425) -> (w431:dbl[])
      }
      frame "数据保存" {
        n221 = flat-sequence {
          tunnel: w456 -> [w462]
          tunnel: w455 -> [w461]
          frame #0 {
            w465 = TRUE ("结束前等待")
            n222 = vi-ref "Calculate&Save.vi"() -> (w459:refnum<vi>)
            n223 = invoke class="VI" method="Ctrl Val.Set"(reference=w459, "Control Name"="机械手" ("控件名"), "Value"=w461) -> (reference out=w460:refnum<vi>)  [unwired: 2 in, 4 out]
            n224 = invoke class="VI" method="Ctrl Val.Set"(reference=w460, "Control Name"="像素" ("控件名"), "Value"=w462) -> (reference out=w468:refnum<vi>)  [unwired: 2 in, 4 out]
            n225 = invoke class="VI" method="FP.Open"(reference=w468, "Activate"=TRUE ("激活？"), "State"=T8."Hidden" ("状态")) -> (reference out=w469:refnum<vi>)  [unwired: 2 in, 4 out]
            n226 = invoke class="VI" method="Run VI"(reference=w469, "Wait until done"=w465, "Auto Dispose Ref"=w465) -> ()  [unwired: 2 in, 5 out]
          }
          frame #1 {
            n227 = One Button Dialog(message="数据保存完成" ("消息"), button name ("OK")="确定" ("按钮名称（“确定”）")) -> ()  [unwired: 1 out]
          }
        }
      }
      frame "退出" {
      }
    }
    n228 = Wait (ms)(milliseconds to wait=u32 50 ("等待时间（毫秒）")) -> ()  [unwired: 1 out]
    n229 = local read "停止标志"() -> (w128:bool)
    n230 = call "Loop.vi"() -> ("Loop Out"=w111:bool)  [unwired: 5 in]
    n231 = Compound Arithmetic op=OR ("复合运算")(w124, w128, w111) -> (w127:bool)
  }
  n232 = invoke class="VI" method="FP.Close"(reference=w13) -> ()  [unwired: 2 in, 3 out]
  n233 = Release Queue(queue=w11, error in (no error)=w12) -> ()  [unwired: 1 in, 3 out]
